vi "Smart Open With Range.vi"(4 "Max Value":dbl[](array[numeric]), 6 "Min Value":dbl[](array[numeric]), 7 "Allow multiple opens?":bool=TRUE, 8 "error in (no error)":errorcluster, 10 "Channel Names":tag[](array[tag])) -> (0 "error out":errorcluster, 3 "AI (N Samples) Ref Out":T1)   [LabVIEW 2021, in "AI Block.lvlib"]
uses:
  <vilib>/myRIO/Instrument Drivers/Onboard IO/AI Block/AI Block.lvlib
  <vilib>/myRIO/Instrument Drivers/Onboard IO/AI Block/vis/myRIO AI N Samples Open.xnode
  <vilib>/myRIO/Common/Instrument Driver Framework/Utilities/typedefs/Analog Scaling Constants.ctl
  <vilib>/myRIO/Common/Instrument Driver Framework/myRIO v1.0/AI Block/typedefs/AI Block Channels Enum.ctl
  <vilib>/myRIO/Common/Instrument Driver Framework/myRIO v1.0/AI Block/typedefs/AI Block Channels List.ctl
  <vilib>/myRIO/Common/Instrument Driver Framework/Utilities/typedefs/Generic FPGA Reference.ctl
  <vilib>/myRIO/Common/Instrument Driver Framework/Utilities/typedefs/myRIO v1.0 Reference.ctl
  <vilib>/myRIO/Common/Instrument Driver Framework/Utilities/typedefs/Hardware Version Enum.ctl
  <vilib>/myRIO/Common/Instrument Driver Framework/Utilities/typedefs/myRIO Generic Hardware Reference.ctl
  <vilib>/myRIO/Instrument Drivers/Onboard IO/AI Block/typedefs/AI Block Reference.ctl
  <vilib>/myRIO/Common/Instrument Driver Framework/ELVIS III v1.0/AI Block/vis/ELVIS III v1.1 Open AI (N Samples).vi
  <vilib>/userdefined/High Color/nirio_resource_hc.ctl
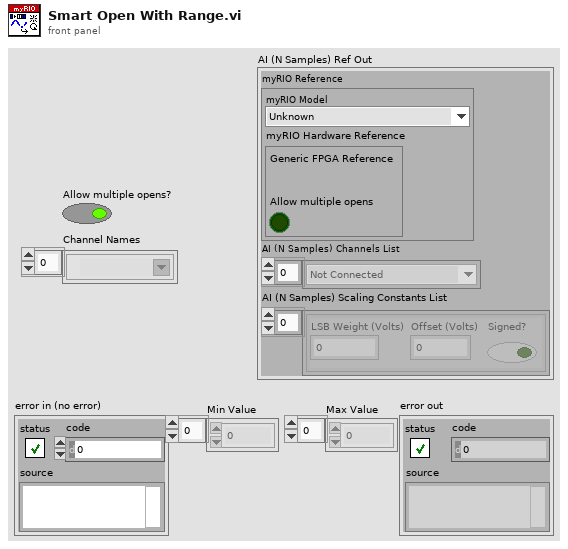
[diagram p1: front panel]
types:
  T1 = typedef "AI Block.lvlib/AI Block Reference.ctl" = cluster{"myRIO Reference":T2, "AI (N Samples) Channels List":T6, "AI (N Samples) Scaling Constants List":T8[]}
  T2 = typedef "myRIO Generic Hardware Reference.ctl" = cluster{"myRIO Model":T3, "myRIO Hardware Reference":T4}
  T3 = typedef "Hardware Version Enum.ctl" = enum16{"Unknown", "myRIO-1900", "myRIO-1950", "roboRIO", "NI ELVIS RIO CM", "ELVIS III"}
  T4 = typedef "myRIO v1.0 Reference.ctl" = cluster{"Generic FPGA Reference":T5, "Allow multiple opens":bool}
  T5 = typedef "Generic FPGA Reference.ctl" = refnum<k20>
  T6 = typedef "AI Block Channels List.ctl" = T7[]
  T7 = typedef "AI Block Channels Enum.ctl" = enum16{"Not Connected", "A/AI0 (N Samples)", "A/AI1 (N Samples)", "A/AI2 (N Samples)", "A/AI3 (N Samples)", "A/AI4 (N Samples)", "A/AI5 (N Samples)", "A/AI6 (N Samples)", "A/AI7 (N Samples)", "A/AI0 (DIFF N Samples)", "A/AI1 (DIFF N Samples)", "A/AI2 (DIFF N Samples)", "A/AI3 (DIFF N Samples)", "B/AI0 (N Samples)", "B/AI1 (N Samples)", "B/AI2 (N Samples)", "B/AI3 (N Samples)", "B/AI4 (N Samples)", "B/AI5 (N Samples)", "B/AI6 (N Samples)", "B/AI7 (N Samples)", "B/AI0 (DIFF N Samples)", "B/AI1 (DIFF N Samples)", "B/AI2 (DIFF N Samples)", "B/AI3 (DIFF N Samples)"}
  T8 = typedef "Analog Scaling Constants.ctl" = cluster{"LSB Weight (Volts)":dbl, "Offset (Volts)":dbl, "Signed?":bool}
  T9 = typedef "nirio_resource_hc.ctl" = tag
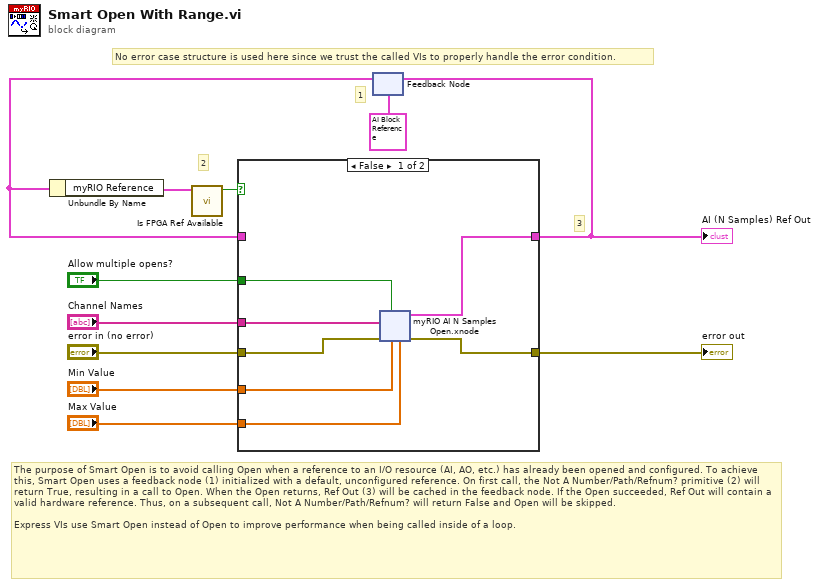
[diagram p0: block diagram]
diagram:
  # "No error case structure is used here since we trust the called VIs to properly handle the error condition."
  # "3"
  # "1"
  # "2"
  # "The purpose of Smart Open is to avoid calling Open when a reference to an I/O resource (AI, AO, etc.) has already been opened and configured. To achieve this, Smart Open uses a feedback node (1) initialized with a default, unconfigured reference. On first call, the Not A Number/Path/Refnum? primitive (2) will return True, resulting in a call to Open. When the Open returns, Ref Out (3) will be cached in the feedback node. If the Open succeeded, Ref Out will contain a valid hardware reference. Thus, on a subsequent call, Not A Number/Path/Refnum? will return False and Open will be skipped.\n\t\nExpress VIs use Smart Open instead of Open to improve performance when being called inside of a loop."
  n1 = feedback #1(T1 {"myRIO Reference"={"myRIO Model"=enum."Unknown", "myRIO Hardware Reference"={"Generic FPGA Reference"=refnum, "Allow multiple opens"=FALSE}}, "AI (N Samples) Channels List"=[], "AI (N Samples) Scaling Constants List"=[]} ("AI Block (N Samples) Ref Out")) -> (w11:T1)
  n2 = Unbundle By Name(w11) -> ("myRIO Reference"=w3:T2)
  n3 = call <vilib>:"Is FPGA Ref Available.vi"("myRIO Reference"=w3) -> ("Is Available?"=w10:bool)  [unwired: 10 in]
  n4 = case shown="False" w10 {
    tunnel: "error in (no error)" -> [w18 w39]
    tunnel: [w17 w40] -> w6
    tunnel: [w16 w39] -> w8
    tunnel: w11 -> [_ w40]
    tunnel: "Channel Names" -> [w14 _]
    tunnel: "Allow multiple opens?" -> [w15 _]
    tunnel: "Min Value" -> [w13 _]
    tunnel: "Max Value" -> [w12 _]
    frame False {
      n5 = xnode "myRIO AI N Samples Open.xnode"("error in (no error)"=w18, "Allow multiple opens?"=w15, "Channel Names"=w14, "Max Value"=w12, "Min Value"=w13) -> ("error out"=w16:errorcluster, "AI (N Samples) Ref Out"=w17:T1)
    }
    frame True {
    }
  }
  "AI (N Samples) Ref Out" <- w6
  "error out" <- w8
  n6 = feedback-in #1(w6) -> ()
